vi "Ruta Inventario--constant.vi"() -> (3 "Ruta Inventario":path)   [LabVIEW 2024, in "ProductControl.lvlib"]
uses:
  ProductControl.lvlib
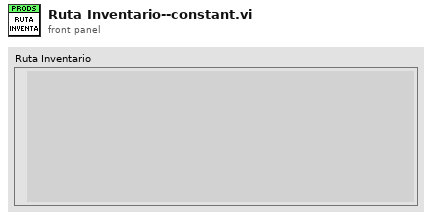
[diagram p1: front panel]
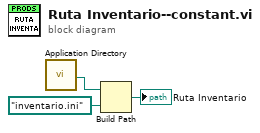
[diagram p0: block diagram]
diagram:
  n1 = call <vilib>:"Application Directory.vi"() -> ("Application Directory"=w1:path)
  n2 = Build Path(base path=w1, name or relative path=path "inventario.ini") -> (appended path=→"Ruta Inventario":path)
